vi "整合命令.vi"(10 "CM":i32, 11 "step":i32) -> (3 "命令":string)   [LabVIEW 2014]
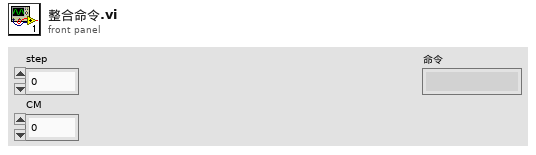
[diagram p1: front panel]
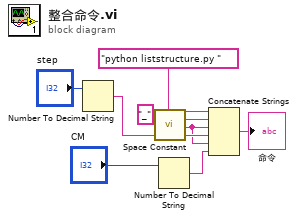
[diagram p0: block diagram]
diagram:
  n1 = Number To Decimal String(number="step") -> (decimal integer string=w8:string)  [unwired: 1 in]
  n2 = call <vilib>:"Space Constant.vi"() -> ("String"=w7:string)
  n3 = Number To Decimal String(number="CM") -> (decimal integer string=w6:string)  [unwired: 1 in]
  n4 = Concatenate Strings("python liststructure.py " ("command line"), "_", w7, w8, w7, w6) -> (→"命令":string)
